vi "MakeChData.vi"(8 "error in (no error)":errorcluster caption="エラー入力（エラーなし）", 10 "サンプリング周期(sec)":dbl, 11 "表 ref":refnum<vi>) -> (0 "error out":errorcluster caption="エラー出力")   [LabVIEW 2014]
uses:
  GlobalData/GlobalData.vi
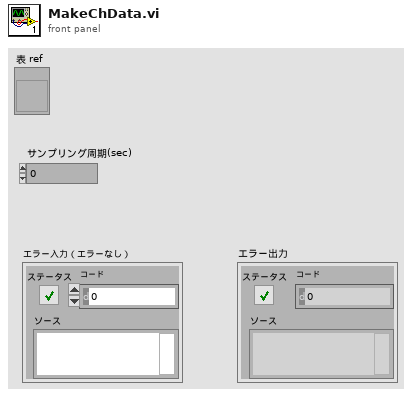
[diagram p1: front panel]
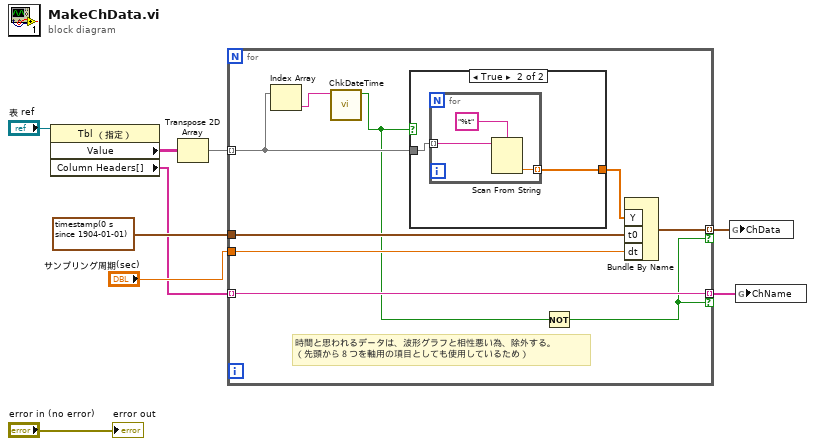
[diagram p0: block diagram]
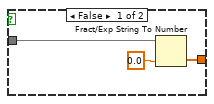
[diagram p2: hidden frame]
diagram:
  n1 = property class="Tbl （指定）"(reference="表 ref") -> ("Value"=w6:string[][], "Column Headers[]"=w1:string[])  [unwired: 1 in, 2 out]
  n2 = Transpose 2D Array(2D array=w6) -> (transposed array=w5:string[][])
  n3 = for {
    tunnel: [w18] -> w9 mode=indexing if=w10
    tunnel: timestamp(0 s since 1904-01-01) ("f") -> [w17]
    tunnel: "サンプリング周期(sec)" -> [w16]
    tunnel: w5 -> [w14] mode=indexing
    tunnel: [w12] -> w2 mode=indexing if=w10
    tunnel: w1 -> [w12] mode=indexing
    # "時間と思われるデータは、波形グラフと相性悪い為、除外する。\n（先頭から８つを軸用の項目としても使用しているため）"
    n4 = Index Array(array=w14) -> (element=w13:string)  [unwired: 1 in]
    n5 = call "ChkDateTime.vi"("文字列"=w13) -> ("ブール"=w11:bool)  [unwired: 10 in]
    n6 = case shown="TRUE" w11 {
      tunnel: w14 -> [w20 w23]
      tunnel: [w19 w22] -> w15
      frame False {
        n7 = Fract/Exp String To Number(string=w20, default (0 dbl)=0.0 ("デフォルト（0 I32）")) -> (number=w19:dbl[])  [unwired: 2 in, 1 out]
      }
      frame True {
        n8 = for {
          tunnel: w23 -> [w25] mode=indexing
          tunnel: [w24] -> w22 mode=indexing
          n9 = Scan From String(format string="%t" ("形式文字列"), input string=w25) -> (output 1=w24:dbl)  [unwired: 3 in, 3 out]
        }
      }
    }
    n10 = Not(x=w11) -> (.not. x?=w10:bool)
    n11 = Bundle By Name("Y"=w15, "t0"=w17, "dt"=w16) -> (w18:waveform(dbl))  [unwired: 1 in]
  }
  n12 = global write "GlobalData.vi" "ChData"(w9) -> ()
  n13 = global write "GlobalData.vi" "ChName"(w2) -> ()
  "error out" <- "error in (no error)"
